vi "testa DH.vi"(0 "VISA Mec":refnum<visa-resource-name>, 2 "string 2":string, 3 "error IO":errorcluster, 4 "destino":T1=enum."fim") -> (5 "Enum":T1, 6 "error out":errorcluster)   [LabVIEW 2011, in "Rotative.lvclass"]
uses:
  Rotative.lvclass
  controls/Enum IC.ctl
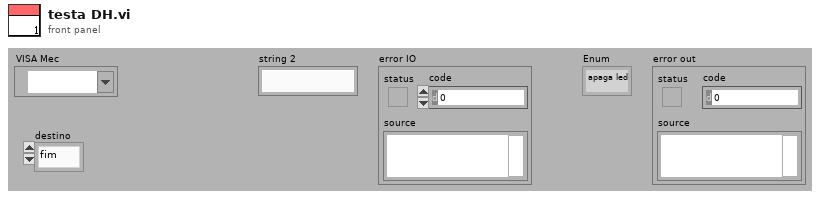
[diagram p1: front panel]
types:
  T1 = typedef "Enum IC.ctl" = enum16{"apaga led", "camera to index", "wait cam index", "grat to index", "wait grat index", "grat to offset", "wait grat off", "grat dh", "cam to offset", "wait cam off", "cam dh", "fim", "erro"}
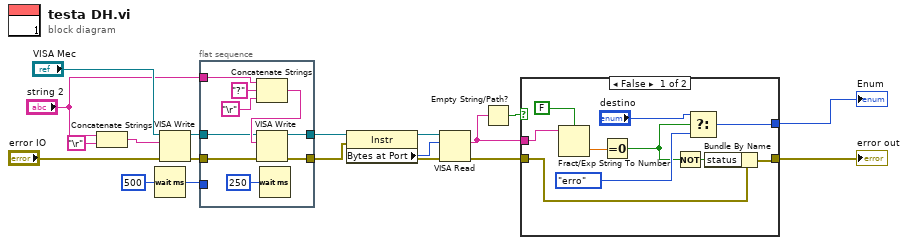
[diagram p0: block diagram]
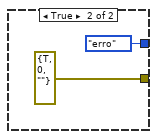
[diagram p2: hidden frame]
diagram:
  n1 = Concatenate Strings("string 2", "\r") -> (w10:string)
  n2 = Wait (ms)(milliseconds to wait=u32 500) -> (millisecond timer value=w15:u32)
  n3 = VISA Write(VISA resource name="VISA Mec", write buffer=w10, error in (no error)="error IO") -> (VISA resource name out=w13:refnum<visa-resource-name>, error out=w11:errorcluster)  [unwired: 1 out]
  n4 = flat-sequence {
    tunnel: w11 -> [w27]
    tunnel: w13 -> [w23]
    tunnel: w15 -> [_]
    tunnel: [w25] -> w16
    tunnel: [w24] -> w17
    tunnel: "string 2" -> [w20]
    frame #0 {
      n5 = Concatenate Strings(w20, "?" ("string"), "\r") -> (w26:string)
      n6 = VISA Write(VISA resource name=w23, write buffer=w26, error in (no error)=w27) -> (VISA resource name out=w25:refnum<visa-resource-name>, error out=w24:errorcluster)  [unwired: 1 out]
      n7 = Wait (ms)(milliseconds to wait=u32 250) -> ()  [unwired: 1 out]
    }
  }
  n8 = property class="Instr"(reference=w16, error in=w17) -> (reference out=w6:refnum<visa-resource-name>, error out=w5:errorcluster, "Bytes at Port"=w4:u32)
  n9 = VISA Read(VISA resource name=w6, byte count=w4, error in (no error)=w5) -> (read buffer=w1:string, error out=w2:errorcluster)  [unwired: 2 out]
  n10 = Empty String/Path?(string/path=w1) -> (empty?=w3:bool)
  n11 = case shown="False" w3 {
    tunnel: w2 -> [w30 _]
    tunnel: [w32 errorcluster {"status"=TRUE, "code"=0, "source"=""} ("error out")] -> w18
    tunnel: w1 -> [w38 _]
    tunnel: [w35 Enum_IC."erro" ("Enum")] -> w19
    frame False {
      n12 = Fract/Exp String To Number(use system decimal point (T)=FALSE, string=w38) -> (number=w36:dbl)  [unwired: 3 out]
      n13 = Equal To 0?(x=w36) -> (x = 0?=w31:bool)
      n14 = Not(x=w31) -> (.not. x?=w29:bool)
      n15 = Select(t="destino", s=w31, f=Enum_IC."erro" ("Enum")) -> (s? t:f=w35:T1)
      n16 = Bundle By Name(cluster=w30, "status"=w29) -> (w32:errorcluster)
    }
    frame True {
    }
  }
  "Enum" <- w19
  "error out" <- w18
